vi "Drive Controller.vi"(8 "error in":errorcluster) -> ()   [LabVIEW 2019]
doc: "This VI executes continuously carrying out the current operation and responding to updates or new operation requests. It will often contain the timing or control code that is difficult to place directly in TeleOp. This VI generally opens all sensors and motors and isolates the rest of the robot code from knowing implementation details of how the operations are carried out."
uses:
  <vilib>/Rock Robotics/WPI/Framework/Completion Status.ctl
  Drive Setpoints.ctl
  Drive Operations.ctl
  Bordeaux/Command Stuff/Single Cmd Info.ctl
  <vilib>/picture/picture.llb/imagedata.ctl
  <vilib>/Rock Robotics/SystemInterfaces/AI/FPGA_AIChannel.ctl
  <vilib>/Rock Robotics/WPI/ThirdParty/REV Robotics/SPARK MAX/Typedef/Spark MAX Control Type.ctl
  <vilib>/Rock Robotics/WPI/Ultrasonic/WPI_SonarMB1010AnalogOpen.vi
  <vilib>/Rock Robotics/WPI/Ultrasonic/WPI_SonarMB1010AnalogGetRange.vi
  Framework/Robot Global Data.vi
panel:
  in  "PID gains M":T1={"proportional gain (Kc)"=0.02, "integral time (Ti, min)"=0.0, "derivative time (Td, min)"=0.0}
  in  "Interactive Values":T2
  in  "Buttons":cluster{"Execute Cmd":bool, "Abort Cmd":bool}
  out "Command Timing":cluster{"Start Time (ms)":u32, "Iterations":i32}
  out "Status":T6
  out "Current\nCmd":string
  # "Tip: The graph shows the motor setpoints. It may also be helpful to observe inputs and sensor values.\nYou may also want to display tuning or debugging controls."
  # "Interactive Command: You may fill in the settings for a command\nand schedule it with the Execute button. You can observe and abort\nany command while fine tuning the code for the controller."
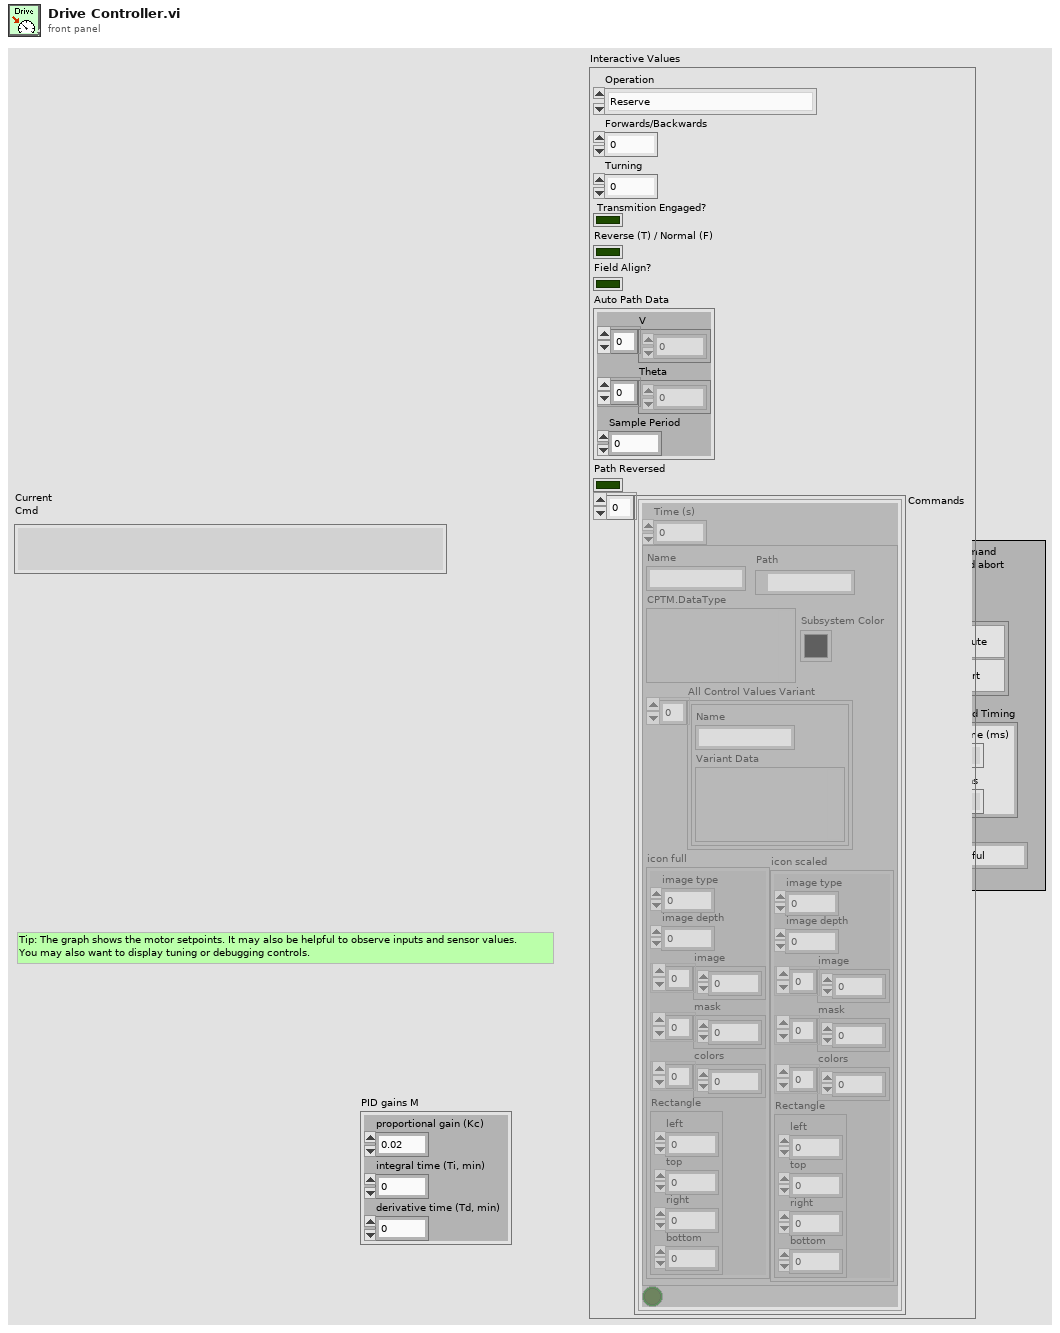
[diagram p1: front panel]
types:
  T1 = cluster{"proportional gain (Kc)":dbl, "integral time (Ti, min)":dbl, "derivative time (Td, min)":dbl}
  T2 = typedef "Drive Setpoints.ctl" = cluster{"Operation":T3, "Forwards/Backwards":dbl, "Turning":dbl, "Transmition Engaged?":bool, "Reverse (T) / Normal (F)":bool, "Field Align?":bool, "Auto Path Data":cluster{"V":dbl[], "Theta":dbl[], "Sample Period":dbl}, "Path Reversed":bool, "Commands":cluster{"Time (s)":dbl, T4, bool}[]}
  T3 = typedef "Drive Operations.ctl" = enum16{"Reserve", "Read Current", "Immediate", "Pod Racer", "Ball AA", "Feeder Station AA", "Play Back From Log"}
  T4 = typedef "Single Cmd Info.ctl" = cluster{"Name":string, "CPTM.DataType":variant, "All Control Values Variant":cluster{"Name":string, "Variant Data":variant}[], "icon full":T5, "icon scaled":T5, "Path":path, "Subsystem Color":u32}
  T5 = typedef "imagedata.ctl" = cluster{"image type":i32, "image depth":i32, "image":u8[], "mask":u8[], "colors":u32[], "Rectangle":cluster{"left":i16, "top":i16, "right":i16, "bottom":i16}}
  T6 = typedef "Completion Status.ctl" = enum16{"Successful", "Aborted", "Incomplete"}
  T7 = cluster{"P Gain":dbl, "I Gain":dbl, "D Gain":dbl, "F Gain":dbl, "I Zone":dbl, "Min Output":dbl, "Max Output":dbl}
  T8 = typedef "FPGA_AIChannel.ctl" = enum8{"AI 0", "AI 1", "AI 2", "AI 3", "AI MXP 0", "AI MXP 1", "AI MXP 2", "AI MXP 3", "Invalid"}
  T9 = typedef "ADIS16448 Device Reference.ctl" = cluster{"DevStatus":errorcluster, "Hardware Config":T10, "Calibration Complete":refnum<notifier>, "Last Value Reference":refnum<data-value>, "Sychronous Process VI":T14, "Cmd FIFO":refnum<k33>, "Source":T15, "IMU Status LED Pin":T12, "Calibration Time":u32}
  T10 = typedef "ADIS16448 Hardware Configuration.ctl" = cluster{"SPI Clock Rate (Hz)":dbl, "IMU SPI Mode (3)":T11, "IMU Reset Pin":T12, "IMU SPI Bus":T13, "IMU Data Ready Pin":T12, "Stall Config":cluster{"Pow2BytesPerRead":u8, "StallTicks":u16, "CsToSclkTicks":u8}, "IMU Status LED Pin":T12}
  T11 = typedef "WPI_SPIMode.ctl" = enum16{"Mode 0 (Clk Idle Low,Sample on Leading)", "Mode 1 (Clk Idle Low,Sample on Trailing)", "Mode 2 (Clk Idle High,Sample on Leading)", "Mode 3 (Clk Idle High,Sample on Trailing)"}
  T12 = typedef "FPGA_DIOChannel.ctl" = enum8{"DIO 0", "DIO 1", "DIO 2", "DIO 3", "DIO 4", "DIO 5", "DIO 6", "DIO 7", "DIO 8", "DIO 9", "DIO MXP 0", "DIO MXP 1", "DIO MXP 2", "DIO MXP 3", "DIO MXP 4", "DIO MXP 5", "DIO MXP 6", "DIO MXP 7", "DIO MXP 8", "DIO MXP 9", "DIO MXP 10", "DIO MXP 11", "DIO MXP 12", "DIO MXP 13", "DIO MXP 14", "DIO MXP 15", "SPI Port CS1", "SPI Port CS2", "SPI Port CS3", "SPI Port MISO", "SPI Port MOSI", "Invalid"}
  T13 = typedef "spi_bus.ctl" = enum16{"SPI On-Board, CS0", "SPI On-Board, CS1", "SPI On-Board, CS2", "SPI On-Board, CS3", "SPI MXP", "Invalid"}
  T14 = typedef "ADIS16448 Process.ctl" = refnum<vi>
  T15 = typedef "FPGA_CounterEncoderSourceConvertionLVSourceType.ctl" = cluster{"DevStatus":errorcluster, "AnalogTriggerMode?":bool, "DigitalMode":cluster{"DIO Channel":T16}, "AnalogTriggerMode":cluster{"AnalogTriggerIndex":T17, "OutputType":T18}}
  T16 = typedef "FPGA_DIODigitalSourceChannel.ctl" = enum8{"DIO 0", "DIO 1", "DIO 2", "DIO 3", "DIO 4", "DIO 5", "DIO 6", "DIO 7", "DIO 8", "DIO 9", "DIO MXP 0", "DIO MXP 1", "DIO MXP 2", "DIO MXP 3", "DIO MXP 4", "DIO MXP 5", "DIO MXP 6", "DIO MXP 7", "DIO MXP 8", "DIO MXP 9", "DIO MXP 10", "DIO MXP 11", "DIO MXP 12", "DIO MXP 13", "DIO MXP 14", "DIO MXP 15", "SPI Port CS1", "SPI Port CS2", "SPI Port CS3", "SPI Port MISO", "SPI Port MOSI", "Disabled"}
  T17 = typedef "FPGA_AnalogTriggerIndex.ctl" = enum8{"Trig 0", "Trig 1", "Trig 2", "Trig 3", "Trig 4", "Trig 5", "Trig 6", "Trig 7", "Invalid"}
  T18 = typedef "FPGA_AnalogTriggerOutType.ctl" = enum16{"InWindow", "TriggerState", "Rising", "Falling"}
  T19 = typedef "WPI_SonarMB1010AnalogDeviceRef.ctl" = cluster{"AIDeviceRef":T20, "Scaling factor (V/in)":dbl, "Average Bits":u8}
  T20 = typedef "WPI_AnalogChannelDevRef.ctl" = cluster{"DevStatus":errorcluster, "Analog Channel":T8}
  T21 = typedef "Command Status Info.ctl" = cluster{"Name":string, "Status":T6, "notifier out":T22}
  T22 = typedef "Completion Notifier.ctl" = refnum<notifier>
  T23 = cluster{"SubSystem Data":T2, cluster{"Start Time (ms)":u32, "Iterations":i32}, cluster{"Command Info":T21, "Description":string, "Default Command":T2, "queue out":refnum<queue>, "Subsystem Name":string}}
  T24 = typedef "Spark MAX Control Type.ctl" = enum16{"Percent VBus", "Voltage", "Velocity", "Position", "Smart Motion", "Current", "Smart Velocity"}
  T25 = enum16{"MAX 90", "Pod Racer", "MAX 180", "Turn to Home", "Turn to Rocket", "Auto-Align", "Turn to ..."}
  T26 = cluster{"V":dbl[], "Theta":dbl[], "Sample Period":dbl}
  T27 = typedef "ADIS16448 Data.ctl" = cluster{"XAngle":dbl, "YAngle":dbl, "ZAngle":dbl}
  T28 = cluster{"SubSystem Data":T2, cluster{"Start Time (ms)":u32, "Iterations":i32}, "Default Command Arguments":cluster{"Command Info":T21, "Description":string, "Default Command":T2, "queue out":refnum<queue>, "Subsystem Name":string}}
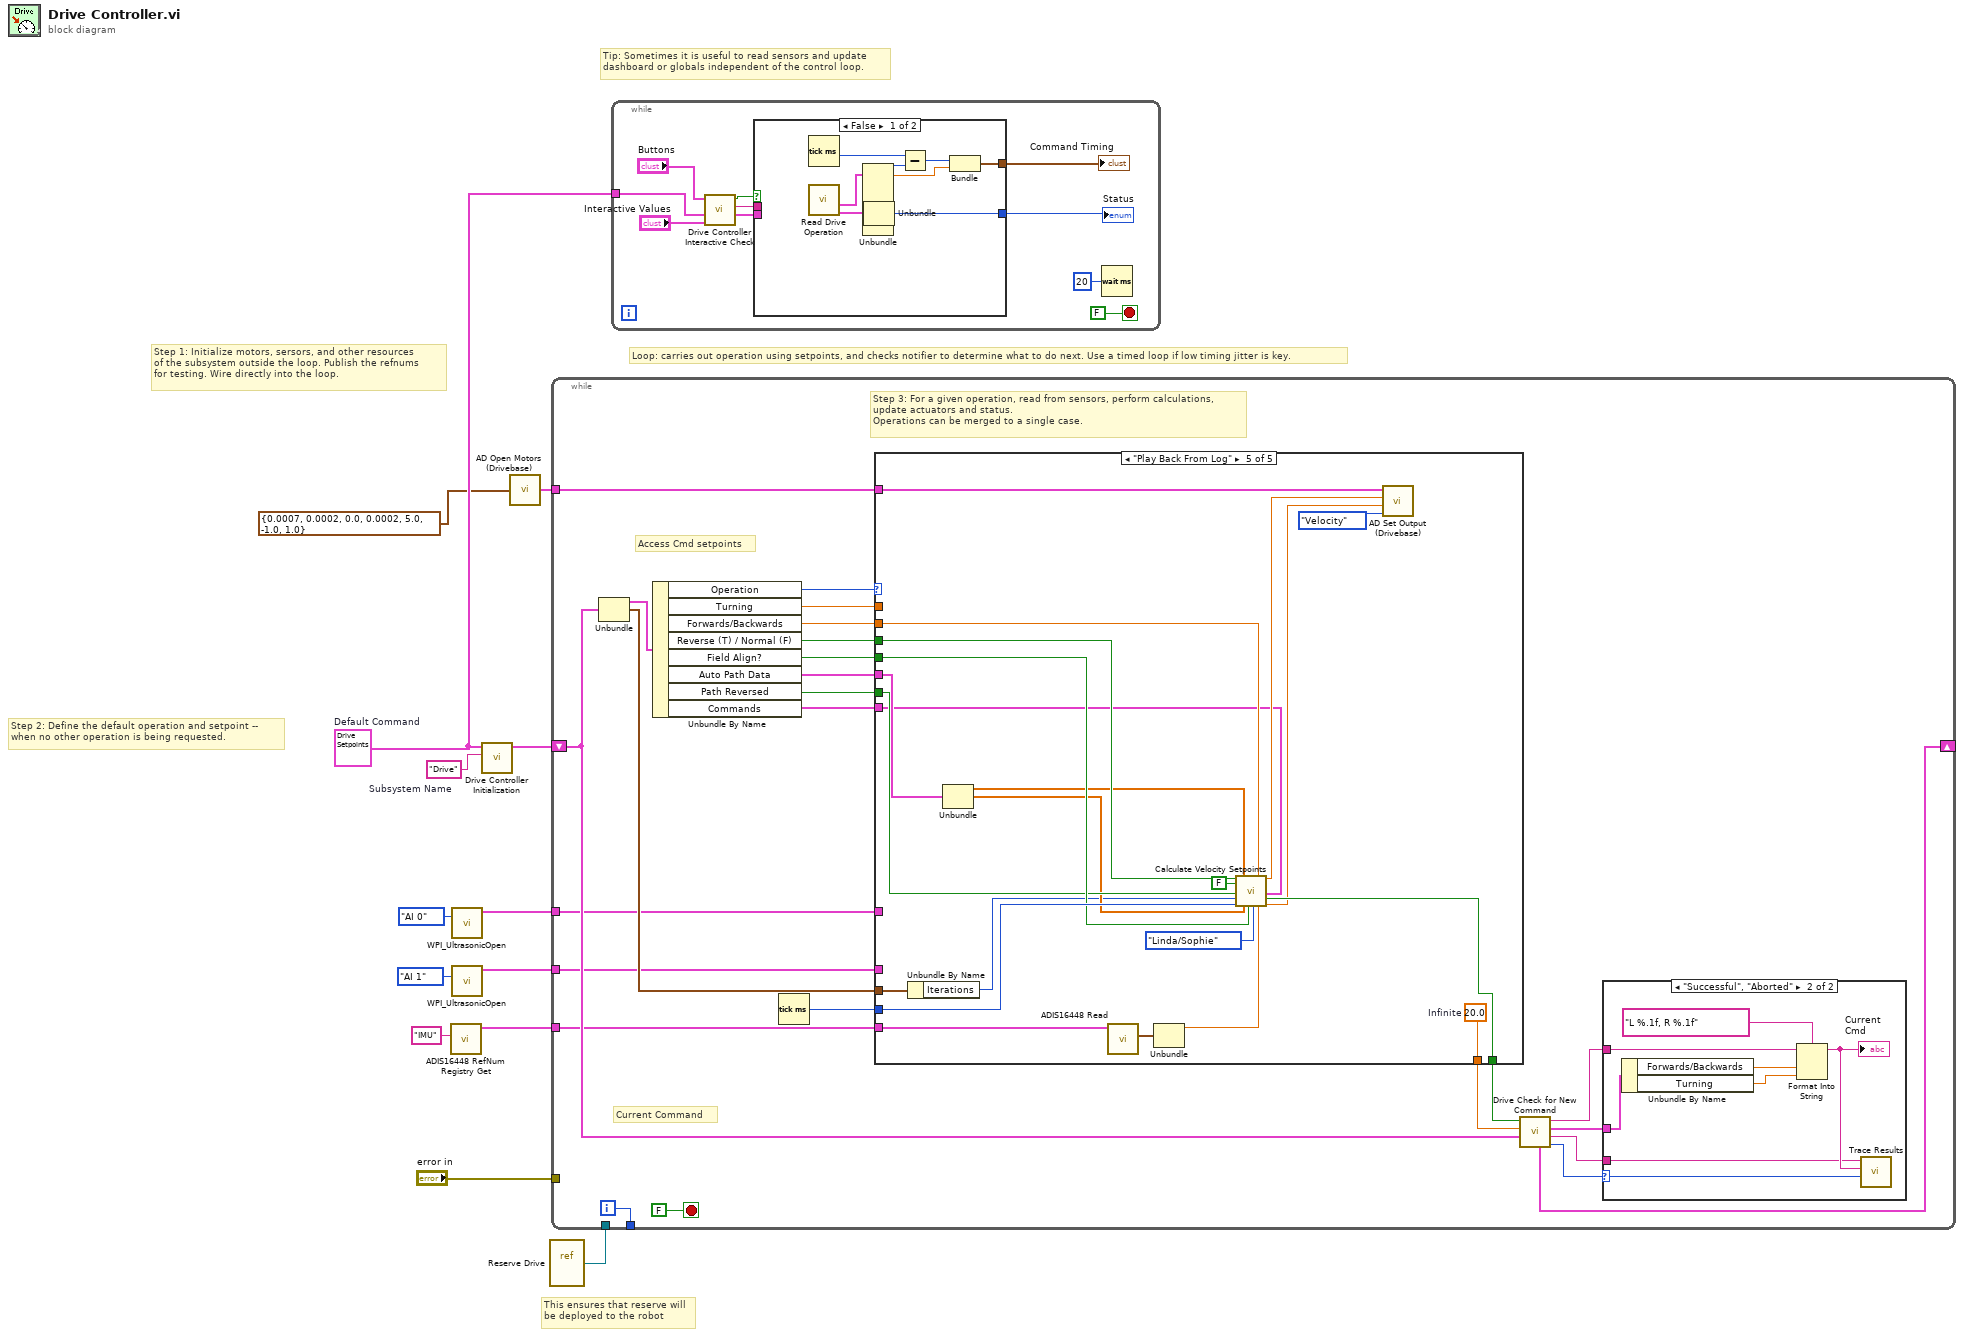
[diagram p0: block diagram]
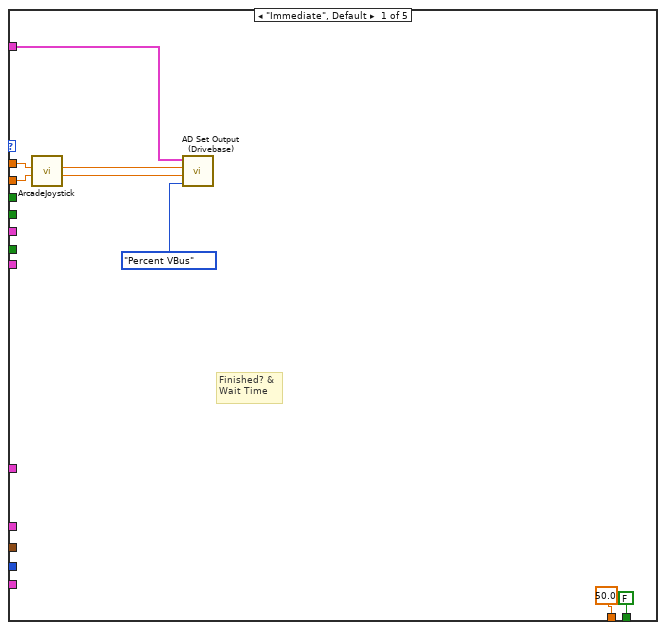
[diagram p2: hidden frame]
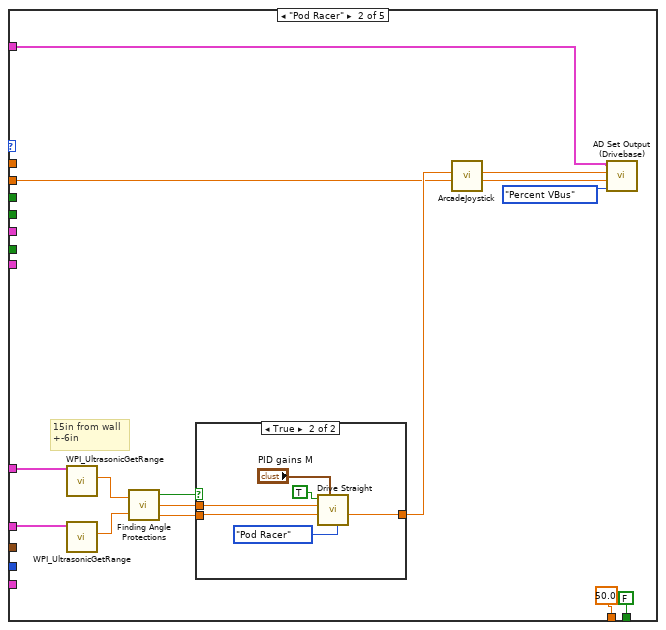
[diagram p3: hidden frame]
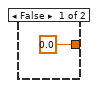
[diagram p4: hidden frame]
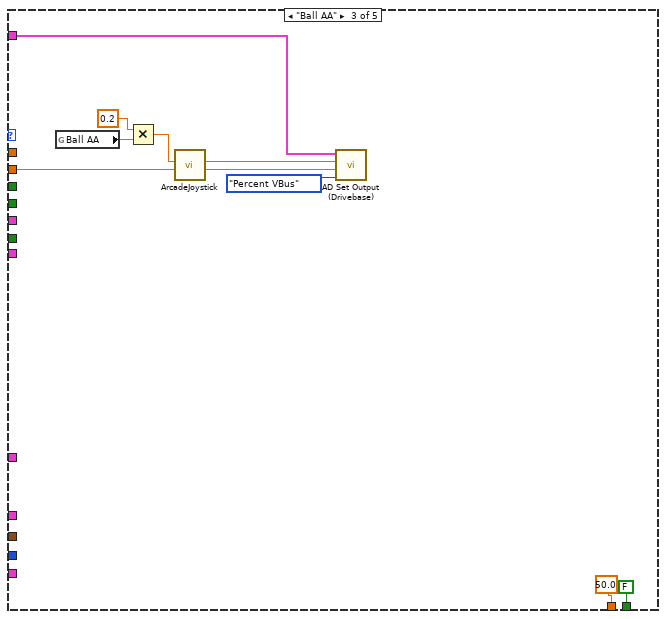
[diagram p5: hidden frame]
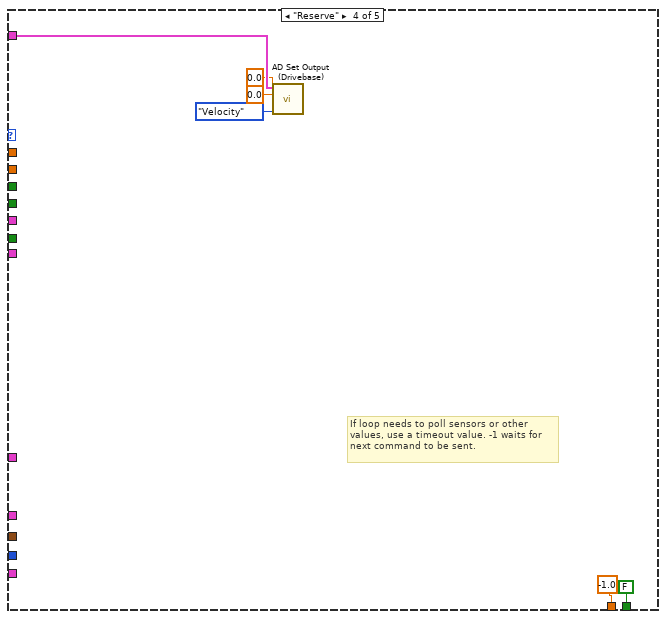
[diagram p6: hidden frame]
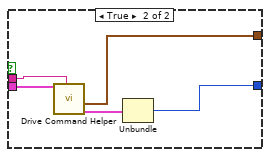
[diagram p8: hidden frame]
diagram:
  w9 = T2 {"Operation"=enum."Reserve", "Forwards/Backwards"=0.0, "Turning"=0.0, "Transmition Engaged?"=FALSE, "Reverse (T) / Normal (F)"=FALSE, "Field Align?"=FALSE, "Auto Path Data"={"V"=[], "Theta"=[], "Sample Period"=0.0}, "Path Reversed"=FALSE, "Commands"=[]}  # Default Command
  w13 = "Drive"  # Subsystem Name
  # "This ensures that reserve will\nbe deployed to the robot"
  # "Tip: Sometimes it is useful to read sensors and update\ndashboard or globals independent of the control loop."
  # "Step 2: Define the default operation and setpoint --\nwhen no other operation is being requested."
  # "Step 1: Initialize motors, sersors, and other resources\nof the subsystem outside the loop. Publish the refnums\nfor testing. Wire directly into the loop."
  # "Loop: carries out operation using setpoints, and checks notifier to determine what to do next. Use a timed loop if low timing jitter is key."
  n1 = call "ADIS16448 RefNum Registry Get.vi"("refnum name"="IMU") -> ("ADIS16448DevRef Out"=w2:T9)  [unwired: 9 in, 1 out]
  n2 = call-poly <vilib>:"WPI_UltrasonicOpen.vi"("Analog Channel"=FPGA_AIChannel."AI 0") -> ("SonarMB1010AnalogDevRef"=w6:T19)  [unwired: 9 in, 1 out]
  n3 = call-poly <vilib>:"WPI_UltrasonicOpen.vi"("Analog Channel"=FPGA_AIChannel."AI 1") -> ("SonarMB1010AnalogDevRef"=w4:T19)  [unwired: 9 in, 1 out]
  n4 = call "Drive Controller Initialization.vi"("Subsystem Name"=w13, "Default Command"=w9) -> ("Current Command"=w11:T23)  [unwired: 9 in]
  n5 = call "AD Open Motors (Drivebase).vi"("PID Constants for Sparks"=T7 {"P Gain"=0.0007, "I Gain"=0.0002, "D Gain"=0.0, "F Gain"=0.0002, "I Zone"=5.0, "Min Output"=-1.0, "Max Output"=1.0}) -> ("output cluster"=w8:cluster{"Left":string[], "Right":string[]})
  n6 = vi-ref "Reserve Drive.vi"() -> (w10:refnum<vi>)
  n7 = while {
    shift-right: [w34] -> _
    shift-left: w11 -> [w30]
    tunnel: [w37] -> _
    tunnel: "error in" -> [_]
    tunnel: w10 -> [_]
    tunnel: w8 -> [w20]
    tunnel: w6 -> [w19]
    tunnel: w4 -> [w18]
    tunnel: w2 -> [w17]
    i -> [w37]
    stop <- FALSE stop-if-true
    # "Current Command"
    # "Access Cmd setpoints"
    # "Step 3: For a given operation, read from sensors, perform calculations,\nupdate actuators and status.\nOperations can be merged to a single case."
    n8 = Unbundle(w30) -> ("SubSystem Data"=w36:T2, w29:cluster{"Start Time (ms)":u32, "Iterations":i32})  [unwired: 1 out]
    n9 = Unbundle By Name(w36) -> ("Operation"=w14:T3, "Turning"=w28:dbl, "Forwards/Backwards"=w27:dbl, "Reverse (T) / Normal (F)"=w26:bool, "Field Align?"=w25:bool, "Auto Path Data"=w24:T26, "Path Reversed"=w23:bool, "Commands"=w22:cluster{"Time (s)":dbl, T4, bool}[])
    n10 = Tick Count (ms)() -> (millisecond timer value=w21:u32)
    n11 = case shown="\"Play Back From Log\"" w14 {
      tunnel: w29 -> [_ _ _ _ w104]
      tunnel: w28 -> [w43 _ _ _ _]
      tunnel: w27 -> [w44 w49 w71 _ w98]
      tunnel: w21 -> [_ _ _ _ w103]
      tunnel: w19 -> [_ w57 _ _ _]
      tunnel: w18 -> [_ w56 _ _ _]
      tunnel: w20 -> [w46 w61 w78 w82 w105]
      tunnel: w26 -> [_ _ _ _ w100]
      tunnel: w25 -> [_ _ _ _ w102]
      tunnel: w23 -> [_ _ _ _ w101]
      tunnel: w24 -> [_ _ _ _ w97]
      tunnel: w22 -> [_ _ _ _ w91]
      tunnel: w17 -> [_ _ _ _ w90]
      tunnel: [FALSE ("Finished?") FALSE ("Finished?") FALSE ("Finished?") FALSE ("Finished?") w88] -> w16
      tunnel: [50.0 ("Infinite") 50.0 ("Infinite") 50.0 ("Infinite") -1.0 ("Infinite") w89] -> w15
      frame "Immediate", Default {
        # "Finished? &\nWait Time"
        n12 = call "ArcadeJoystick.vi"("Y axis value"=w44, "X axis value"=w43) -> ("Right Motor Value"=w39:dbl, "Left Motor Value"=w40:dbl)  [unwired: 8 in]
        n13 = call "AD Set Output (Drivebase).vi"("Control Mode"=Spark_MAX_Control_Type."Percent VBus", "Right"=w39, "Left"=w40, "Input cluster"=w46) -> ()  [unwired: 2 in]
      }
      frame "Pod Racer" {
        # "15in from wall\n+-6in"
        n14 = call-poly <vilib>:"WPI_UltrasonicGetRange.vi"("SonarMB1010AnalogDevRef"=w57) -> ("Distance"=w54:dbl)  [unwired: 8 in, 2 out]
        n15 = call-poly <vilib>:"WPI_UltrasonicGetRange.vi"("SonarMB1010AnalogDevRef"=w56) -> ("Distance"=w53:dbl)  [unwired: 8 in, 2 out]
        n16 = call "Finding Angle Protections.vi"("Distance 1"=w54, "Distance 2"=w53) -> ("Trigger?"=w52:bool, "Angle to Turn"=w51:dbl, "Current Angle"=w50:dbl)
        n17 = case shown="True" w52 {
          tunnel: [0.0 ("Turn Setpoint") w68] -> w55
          tunnel: w51 -> [_ w64]
          tunnel: w50 -> [_ w63]
          frame False {
          }
          frame True {
            n18 = call "Drive Straight.vi"("Maneuver"=T25."Pod Racer", "PID gains M"="PID gains M", "Angle"=w63, "Angle to Get"=w64, "Enable?"=TRUE) -> ("Turn Setpoint"=w68:dbl)  [unwired: 6 in]
          }
        }
        n19 = call "ArcadeJoystick.vi"("Y axis value"=w49, "X axis value"=w55) -> ("Right Motor Value"=w59:dbl, "Left Motor Value"=w60:dbl)  [unwired: 8 in]
        n20 = call "AD Set Output (Drivebase).vi"("Control Mode"=Spark_MAX_Control_Type."Percent VBus", "Right"=w59, "Left"=w60, "Input cluster"=w61) -> ()  [unwired: 2 in]
      }
      frame "Ball AA" {
        n21 = global read "Robot Global Data.vi" "Ball AA"() -> (w74:dbl)
        n22 = Multiply(x=0.2, y=w74) -> (x*y=w72:dbl)
        n23 = call "ArcadeJoystick.vi"("Y axis value"=w71, "X axis value"=w72) -> ("Right Motor Value"=w75:dbl, "Left Motor Value"=w77:dbl)  [unwired: 8 in]
        n24 = call "AD Set Output (Drivebase).vi"("Control Mode"=Spark_MAX_Control_Type."Percent VBus", "Right"=w75, "Left"=w77, "Input cluster"=w78) -> ()  [unwired: 2 in]
      }
      frame "Reserve" {
        # "If loop needs to poll sensors or other\nvalues, use a timeout value. -1 waits for\nnext command to be sent."
        n25 = call "AD Set Output (Drivebase).vi"("Control Mode"=Spark_MAX_Control_Type."Velocity", "Right"=0.0, "Left"=0.0, "Input cluster"=w82) -> ()  [unwired: 2 in]
      }
      frame "Play Back From Log" {
        w89 = 20.0  # Infinite
        n26 = Unbundle By Name(w104) -> ("Iterations"=w86:i32)
        n27 = Unbundle(w97) -> ("V"=w96:dbl[], "Theta"=w95:dbl[])  [unwired: 1 out]
        n28 = call "ADIS16448 Read.vi"("ADIS16448DevRef"=w90) -> ("Gyro Value"=w93:T27)  [unwired: 3 in, 7 out]
        n29 = Unbundle(w93) -> ("XAngle"=w87:dbl)  [unwired: 2 out]
        n30 = call "Calculate Velocity Setpoints.vi"("Negated"=w100, "Front is Back"=FALSE, "Reversed"=w101, "Iterations"=w86, "Time"=w103, "Velocity Data"=w96, "Angular Data (Relative)"=w95, "Align?"=w102, "Enum"=enum16{"Vantage", "Mule", "Linda/Sophie"}."Linda/Sophie", "Angle To Get"=w98, "IMU Input"=w87, "Commands"=w91) -> ("Left Setpoint"=w106:dbl, "Finished?"=w88:bool, "Right Setpoint"=w85:dbl)  [unwired: 3 in, 2 out]
        n31 = call "AD Set Output (Drivebase).vi"("Control Mode"=Spark_MAX_Control_Type."Velocity", "Right"=w85, "Left"=w106, "Input cluster"=w105) -> ()  [unwired: 2 in]
      }
    }
    n32 = call "Drive Check for New Command.vi"("input cluster"=w30, "Wait time (ms)"=w15, "Finished?"=w16) -> ("Completion"=w35:T6, "Subsystem Name"=w31:string, "Current Command"=w32:T2, "Initial Trace String"=w33:string, "Next Command"=w34:T28)  [unwired: 4 in]
    n33 = case shown="\"Successful\", \"Aborted\"" w35 {
      selector: w35 -> [_ w114]
      tunnel: w33 -> [_ w109]
      tunnel: w32 -> [_ w110]
      tunnel: w31 -> [_ w107]
      frame "Incomplete", Default {
        # "Continuing current command"
      }
      frame "Successful", "Aborted" {
        # "Report and setup for next command"
        n34 = Unbundle By Name(w110) -> ("Forwards/Backwards"=w112:dbl, "Turning"=w113:dbl)
        n35 = Format Into String(format string="L %.1f, R %.1f", initial string=w109, w112, w113) -> (resulting string=w108:string)  [unwired: 1 in, 1 out]
        "Current\nCmd" <- w108
        n36 = call <vilib>:"Trace Results.vi"("Status of previous command"=w114, "Description"=w108, "Subsystem"=w107) -> ()  [unwired: 9 in]
      }
    }
  }
  n37 = while {
    tunnel: w9 -> [w116]
    stop <- FALSE stop-if-true
    n38 = call "Drive Controller Interactive Check.vi"("Interactive Command In"="Interactive Values", "Default Command"=w116, "Buttons"="Buttons") -> ("Interactive Command Out"=w118:T2, "Trace String"=w119:string, "Schedule"=w120:bool)  [unwired: 6 in]
    n39 = case shown="False" w120 {
      tunnel: [w129 w137] -> w121
      tunnel: [w128 w133] -> w122
      tunnel: w119 -> [_ w135]
      tunnel: w118 -> [_ w134]
      frame False {
        n40 = Tick Count (ms)() -> (millisecond timer value=w132:u32)
        n41 = call "Read Drive Operation.vi"() -> ("Command Info"=w126:T21, "SubSystem Data"=w125:T2)  [unwired: 9 in, 1 out]
        n42 = Unbundle(w125) -> ("Operation"=w130:T3, "Forwards/Backwards"=w127:dbl)  [unwired: 7 out]
        n43 = Unbundle(w126) -> ("Status"=w129:T6)  [unwired: 2 out]
        n44 = Subtract(x=w132, y=w130) -> (x-y=w131:u32)
        n45 = Bundle(w131, "Forwards/Backwards"=w127) -> (w128:cluster{u32, "Forwards/Backwards":dbl})  [unwired: 1 in]
      }
      frame True {
        n46 = call "Drive Command Helper.vi"("Description"=w135, "SubSystem Data"=w134) -> ("Command Info Out"=w136:T21, "Command Timing"=w133:cluster{"Start Time (ms)":u32, "Iterations":i32})  [unwired: 7 in, 1 out]
        n47 = Unbundle(w136) -> ("Status"=w137:T6)  [unwired: 2 out]
      }
    }
    "Status" <- w121
    "Command Timing" <- w122
    n48 = Wait (ms)(milliseconds to wait=u32 20) -> ()  [unwired: 1 out]
  }
